vi "LDC-37X4C Set Laser Current Limits.vi"(8 "error in (no error)":errorcluster, 10 "Limit":i32=500, 11 "VISA resource name":refnum<visa-resource-name>) -> (0 "error out":errorcluster, 3 "VISA resource name out":refnum<visa-resource-name>)   [LabVIEW 2021]
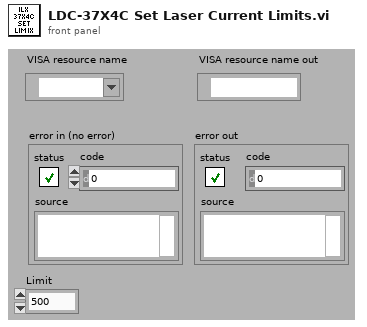
[diagram p1: front panel]
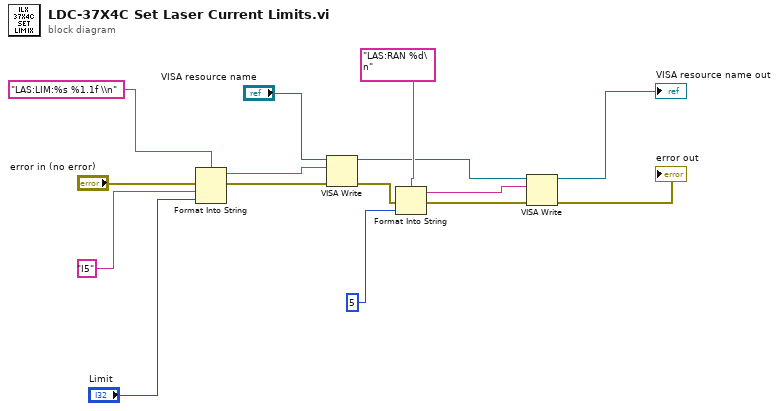
[diagram p0: block diagram]
diagram:
  n1 = Format Into String(format string="LAS:LIM:%s %1.1f \\n", error in="error in (no error)", "I5" ("input 1"), "Limit") -> (resulting string=w14:string, error out=w12:errorcluster)  [unwired: 1 in]
  n2 = VISA Write(VISA resource name="VISA resource name", write buffer=w14, error in (no error)=w12) -> (VISA resource name out=w4:refnum<visa-resource-name>, error out=w3:errorcluster)  [unwired: 1 out]
  n3 = Format Into String(format string="LAS:RAN %d\n", error in=w3, 5 ("Range")) -> (resulting string=w8:string, error out=w7:errorcluster)  [unwired: 1 in]
  n4 = VISA Write(VISA resource name=w4, write buffer=w8, error in (no error)=w7) -> (VISA resource name out=→"VISA resource name out":refnum<visa-resource-name>, error out=→"error out":errorcluster)  [unwired: 1 out]
